vi "_PC_D999_upd_user_param.vi"(7 "refnum cluster":T1, 8 "error in (no error)":errorcluster, 11 "D999_Param":T2={"Enable"=FALSE, "AI"=[{"Label"="", "MultiValue"=1.0, "AddValue"=0.0}, {"Label"="", "MultiValue"=1.0, "AddValue"=0.0}, {"Label"="", "MultiValue"=1.0, "AddValue"=0.0}, {"Label"="", "MultiValue"=1.0, "AddValue"=0.0}, {"Label"="", "MultiValue"=1.0, "AddValue"=0.0}, {"Label"="", "MultiValue"=1.0, "AddValue"=0.0}, {"Label"="", "MultiValue"=1.0, "AddValue"=0.0}, {"Label"="", "MultiValue"=1.0, "AddValue"=0.0}, {"Label"="", "MultiValue"=1.0, "AddValue"=0.0}, {"Label"="", "MultiValue"=1.0, "AddValue"=0.0}, {"Label"="", "MultiValue"=1.0, "AddValue"=0.0}, {"Label"="", "MultiValue"=1.0, "AddValue"=0.0}], "AO"=[], "Switch"=[]}) -> (0 "error out":errorcluster)   [LabVIEW 2018]
uses:
  RT/PublicSubVI/Ctl/_ctl_RT_D999_Param.ctl
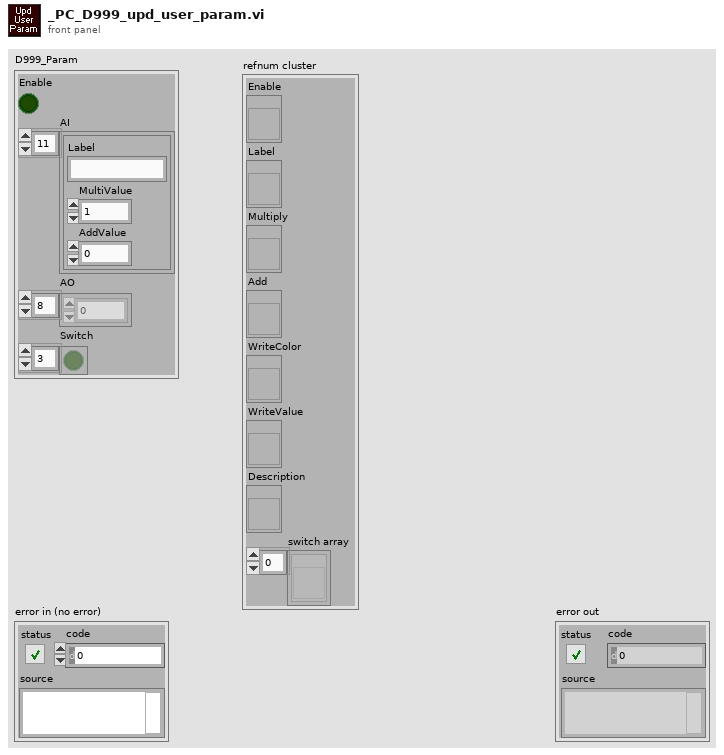
[diagram p1: front panel]
types:
  T1 = cluster{"Enable":refnum<vi>, "Label":refnum<vi>, "Multiply":refnum<vi>, "Add":refnum<vi>, "WriteColor":refnum<vi>, "WriteValue":refnum<vi>, "Description":refnum<vi>, "switch array":refnum<vi>[]}
  T2 = typedef "_ctl_RT_D999_Param.ctl" = cluster{"Enable":bool, "AI":cluster{"Label":string, "MultiValue":dbl, "AddValue":dbl}[], "AO":i16[], "Switch":bool[]}
  T3 = cluster{"Label":string, "MultiValue":dbl, "AddValue":dbl}[]
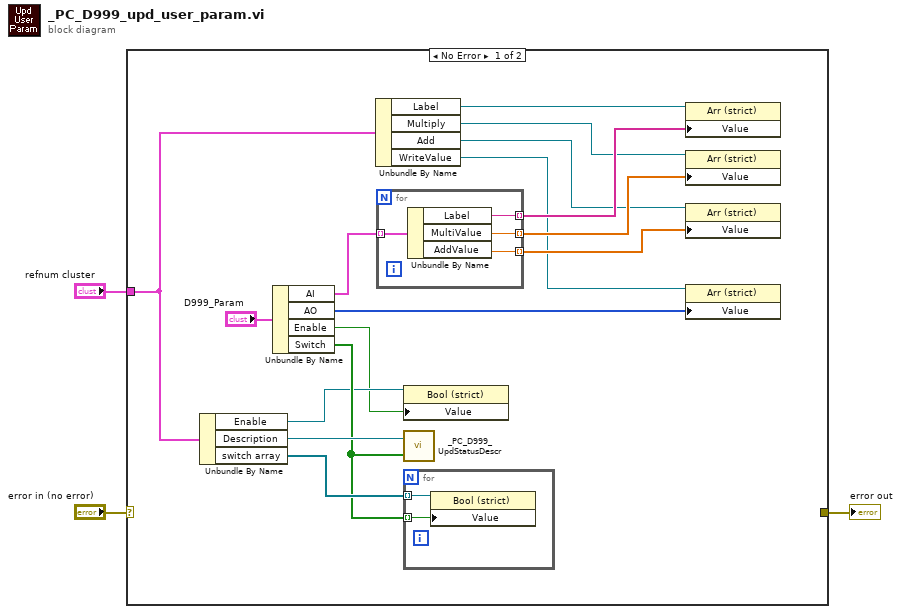
[diagram p0: block diagram]
diagram:
  n1 = case shown="No Error" "error in (no error)" {
    selector: "error in (no error)" -> [_ w26]
    tunnel: [_ w26] -> w2
    tunnel: "refnum cluster" -> [w9 _]
    frame No Error {
      n2 = Unbundle By Name(w9) -> ("Enable"=w5:refnum<vi>, "Description"=w8:refnum<vi>, "switch array"=w7:refnum<vi>[])
      n3 = Unbundle By Name("D999_Param") -> ("AI"=w18:T3, "AO"=w10:i16[], "Enable"=w4:bool, "Switch"=w6:bool[])
      n4 = Unbundle By Name(w9) -> ("Label"=w17:refnum<vi>, "Multiply"=w15:refnum<vi>, "Add"=w13:refnum<vi>, "WriteValue"=w11:refnum<vi>)
      n5 = for {
        tunnel: w18 -> [w25] mode=indexing
        tunnel: [w24] -> w16 mode=indexing
        tunnel: [w23] -> w14 mode=indexing
        tunnel: [w22] -> w12 mode=indexing
        n6 = Unbundle By Name(w25) -> ("Label"=w24:string, "MultiValue"=w23:dbl, "AddValue"=w22:dbl)
      }
      n7 = property class="Bool (strict)"(reference=w5, "Value"=w4) -> ()  [unwired: 1 in, 2 out]
      n8 = call "_PC_D999_UpdStatusDescr.vi"("Switch Enable"=w6, "Description"=w8) -> ()  [unwired: 1 in]
      n9 = for {
        tunnel: w7 -> [w21] mode=indexing
        tunnel: w6 -> [w20] mode=indexing
        n10 = property class="Bool (strict)"(reference=w21, "Value"=w20) -> ()  [unwired: 1 in, 2 out]
      }
      n11 = property class="Arr (strict)"(reference=w17, "Value"=w16) -> ()  [unwired: 1 in, 2 out]
      n12 = property class="Arr (strict)"(reference=w15, "Value"=w14) -> ()  [unwired: 1 in, 2 out]
      n13 = property class="Arr (strict)"(reference=w13, "Value"=w12) -> ()  [unwired: 1 in, 2 out]
      n14 = property class="Arr (strict)"(reference=w11, "Value"=w10) -> ()  [unwired: 1 in, 2 out]
    }
    frame Error {
    }
  }
  "error out" <- w2
